vi "SevenSegmentDisplay.vi"() -> ()   [LabVIEW 2019]
panel:
  in  "stop":bool
  in  "Number":u8
  out "e":bool
  out "f":bool
  out "c":bool
  out "g":bool
  out "b":bool
  out "d":bool
  out "a":bool
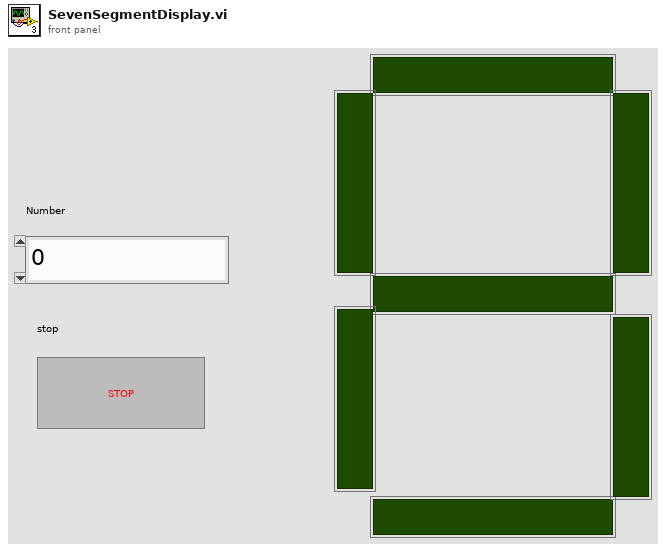
[diagram p1: front panel]
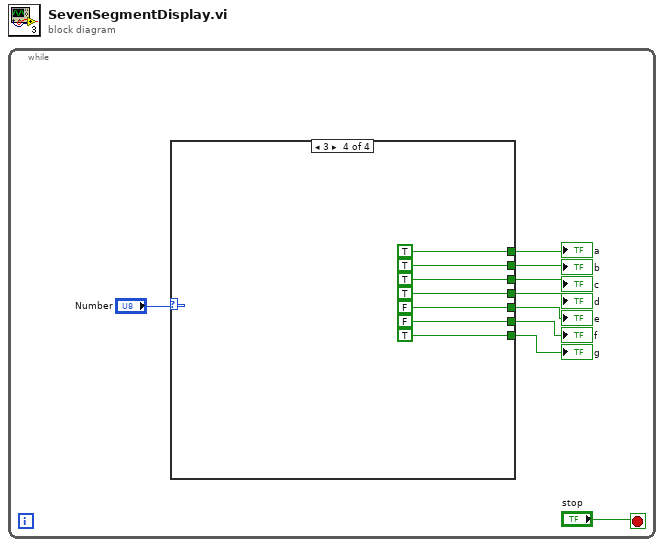
[diagram p0: block diagram]
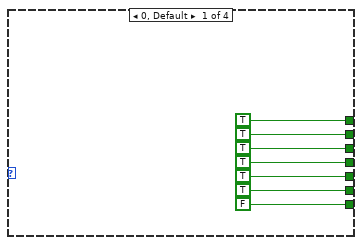
[diagram p2: hidden frame]
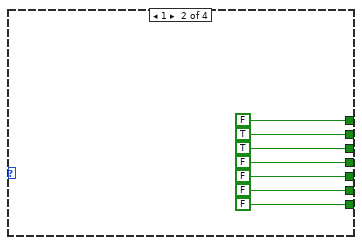
[diagram p3: hidden frame]
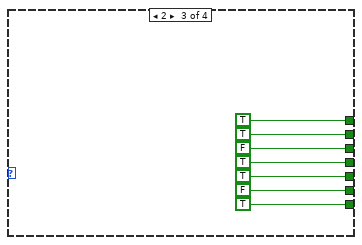
[diagram p4: hidden frame]
diagram:
  n1 = while {
    stop <- "stop" stop-if-true
    n2 = case shown="3" "Number" {
      tunnel: [TRUE FALSE TRUE TRUE] -> w8
      tunnel: [TRUE TRUE TRUE TRUE] -> w7
      tunnel: [TRUE TRUE FALSE TRUE] -> w6
      tunnel: [TRUE FALSE TRUE TRUE] -> w5
      tunnel: [TRUE FALSE TRUE FALSE] -> w4
      tunnel: [TRUE FALSE FALSE FALSE] -> w3
      tunnel: [FALSE FALSE TRUE TRUE] -> w2
      frame 0, Default {
      }
      frame 1 {
      }
      frame 2 {
      }
      frame 3 {
      }
    }
    "a" <- w8
    "d" <- w5
    "b" <- w7
    "g" <- w2
    "c" <- w6
    "f" <- w3
    "e" <- w4
  }
